vi "SpeakerTask.vi"(0 "stop":bool, 3 "ChanSelect":enum16{"Left", "Right", "Stereo"}(ring), 4 "path":path=path "E:/Code/Labview/SoundIdentity/Sounds/Test/TestANJALI.wav") -> (1 "Waveform Graph":waveform(dbl)[](graph)=[{"t0"=timestamp(0 s since 1904-01-01), "dt"=6.25e-05, "Y"=array[16640 elements]}])   [LabVIEW 2010]
doc: "I. Description:\nThis example demonstrates how to output a continuous periodic waveform using an internal sample clock.\n\nII. Instructions for Running:\n1. Select the Physical Channel to correspond to where your signal is output on the DAQ device.\n2. Enter the Minimum and Maximum Voltage Ranges\n3. Specify the Desired Frequency of the output Waveform\n4. Enter the Waveform Information. See the documentation of the Waveform Buffer Generation SubVI for information on each parameter.\n\nIII. Block Diagram Steps:\n1. Create an Analog Output Voltage channel.\n2. Call the DAQmx Timing (Use Waveform) VI which sets the sample clock rate based on the input waveform parameters, and set the sample mode to Continuous.\n3. Write the waveform to the output buffer.\n4. Call the Start VI.\n5. Loop continuously until the user presses the Stop button. Check for errors every 100 ms using the Is Task Done? VI\n6. Clear the Task\n7. Use the popup dialog box to display an error or warning if any.\n\nIV. I/O Connections Overview:\nMake sure your signal output terminal matches the Physical Channel I/O Control. For further connection information, refer to your hardware reference manual."
uses:
  <vilib>/Utility/error.llb/DialogType.ctl
  <vilib>/DAQmx/write.llb/DAQmx Write (Analog 2D DBL NChan NSamp).vi
  <vilib>/DAQmx/configure/timing.llb/DAQmx Timing (Sample Clock).vi
  <vilib>/measure/maspectr.llb/FFT Power Spectrum for N Chan.vi
  <vilib>/daqmx/miscellaneous.llb/DAQmx Fill In Error Info.vi
  <vilib>/DAQmx/create/channels.llb/DAQmx Create Channel (AO-Voltage-Basic).vi
  <vilib>/measure/NI_MAPro.lvlib
panel:
  in  "Power Spectrum":bool
  out "Power Spectrum 2":cluster{"f0":dbl, "df":dbl, "magnitude":dbl[]}[](graph)
  out "Done":bool=TRUE
  out "Completed":dbl=1.0 format="%0.0f"
  in  "restart":bool
  in  "dB":bool=TRUE
  in  "stop 2":bool
  in  "window":T1(ring)=enum."Hanning"
  in  "averaging parameters":T2={"averaging mode"=enum."No averaging", "weighting mode"=enum."Exponential", "number of averages"=10} {"number of averages" min=1}
  in  "Minimum Value":dbl=-10.0 format="%0.2f"
  in  "Maximum Value":dbl=10.0 format="%0.2f"
  # "Real-Time Spectral Measurements"
  # "Sampling Rate"
  # "Wav File"
  # "Channel Parameters"
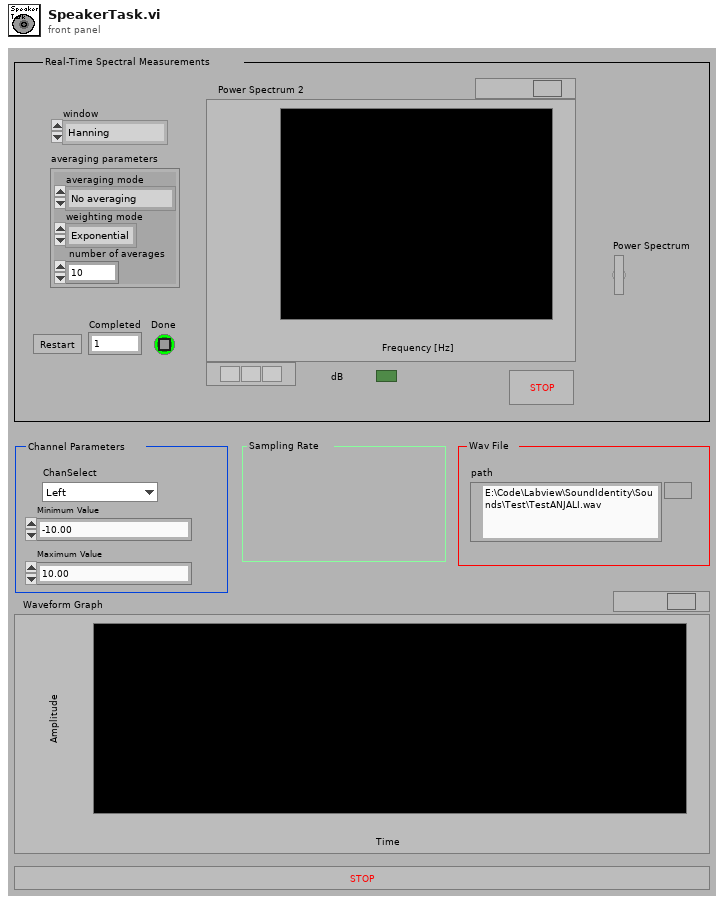
[diagram p1: front panel]
types:
  T1 = enum16{"None ", "Hanning", "Hamming", "Blackman-Harris", "Exact Blackman", "Blackman", "Flat Top", "4 Term B-Harris ", "7 Term B-Harris", "Low Sidelobe"}
  T2 = cluster{"averaging mode":enum16{"No averaging", "Vector averaging", "RMS averaging", "Peak hold"}, "weighting mode":enum16{"Linear", "Exponential"}, "number of averages":u32}
  T3 = typedef "DialogType.ctl" = u16
  T4 = cluster{"data[0]":waveform(dbl), "data[1]":waveform(dbl), "data[2]":waveform(dbl), "data[3]":waveform(dbl), "data[4]":waveform(dbl), "data[5]":waveform(dbl), "data[6]":waveform(dbl), "data[7]":waveform(dbl), "data[8]":waveform(dbl)}
  T5 = enum16{"Initialize", "String", "Start", "New Session", "Stop", "Resume", "Close"}
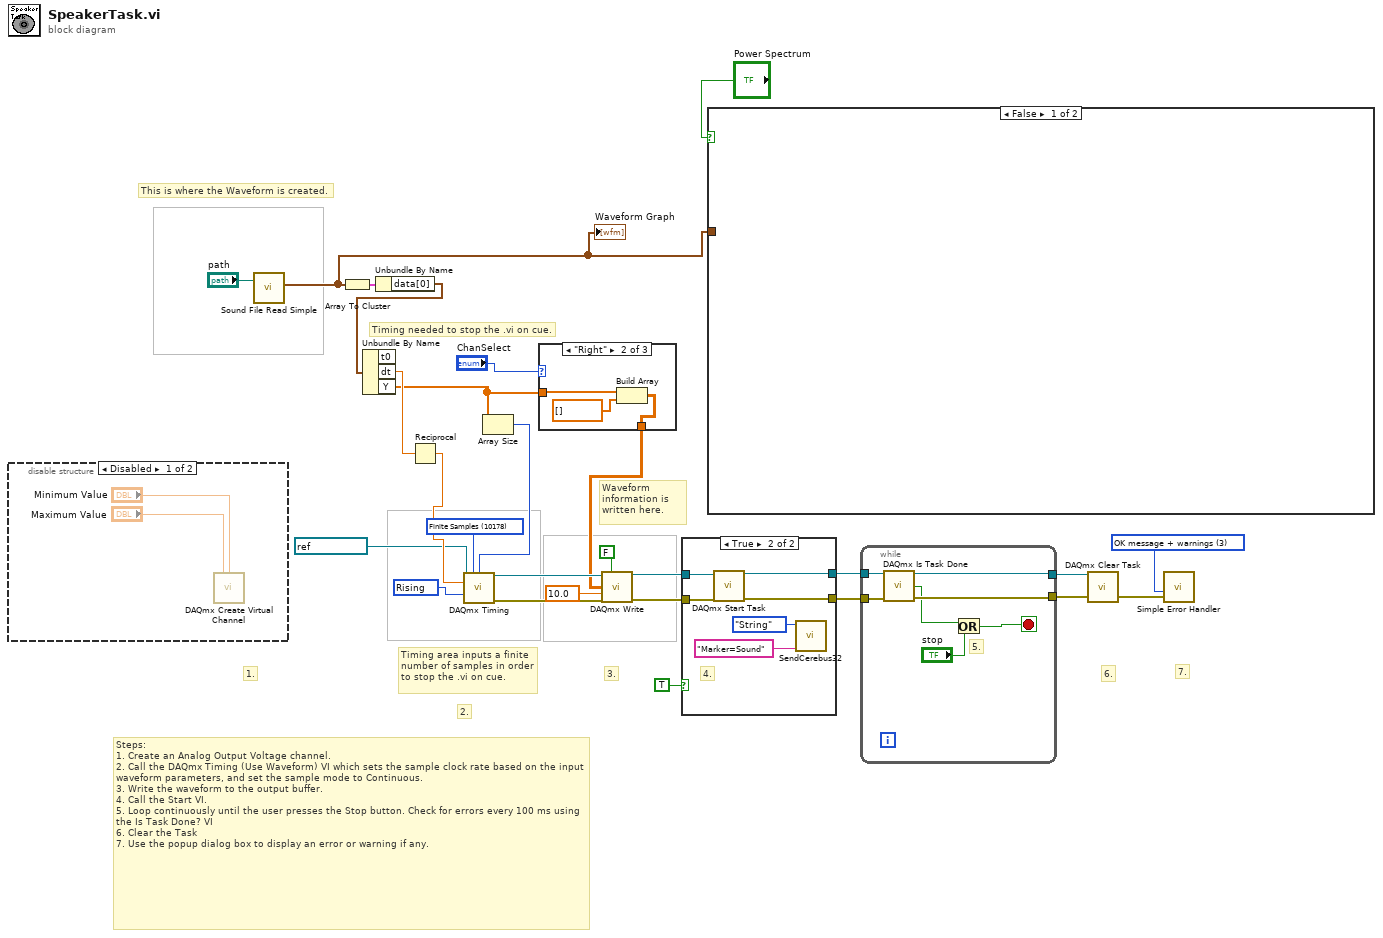
[diagram p0: block diagram]
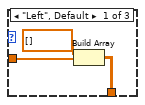
[diagram p2: hidden frame]
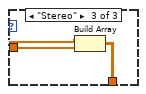
[diagram p3: hidden frame]
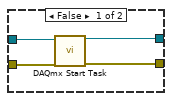
[diagram p5: hidden frame]
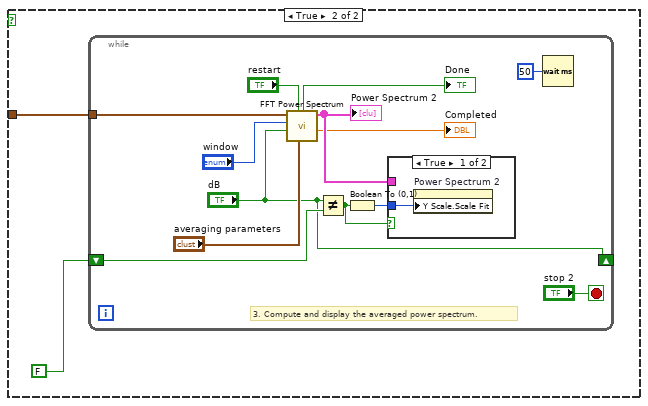
[diagram p6: hidden frame]
diagram:
  w15 = 10280 items=["Rising"=10280, "Falling"=10171] ("active edge")
  w18 = T3 3 items=["no dialog", "OK message", "continue or stop message", "OK message + warnings", "continue/stop + warnings"] ("type of dialog (OK msg:1)")
  w26 = 10178 items=["Finite Samples"=10178, "Continuous Samples"=10123] ("sample mode")
  # "Waveform information is written here."
  # "Timing area inputs a finite number of samples in order to stop the .vi on cue."
  # "Timing needed to stop the .vi on cue."
  # "This is where the Waveform is created."
  # "7."
  # "6."
  # "Steps: \n1. Create an Analog Output Voltage channel.\n2. Call the DAQmx Timing (Use Waveform) VI which sets the sample clock rate based on the input waveform parameters, and set the sample mode to Continuous.\n3. Write the waveform to the output buffer.\n4. Call the Start VI.\n5. Loop continuously until the user presses the Stop button. Check for errors every 100 ms using the Is Task Done? VI\n6. Clear the Task\n7. Use the popup dialog box to display an error or warning if any."
  # "3."
  # "2."
  # "1."
  n1 = disable-structure shown="Disabled" {
    frame Disabled {
      n2 = call-poly <vilib>:"DAQmx Create Virtual Channel.vi"("maximum value"="Maximum Value", "minimum value"="Minimum Value") -> ()  [unwired: 12 in, 2 out]
    }
    frame Enabled {
    }
  }
  n3 = call <vilib>:"Sound File Read Simple.vi"("path"="path") -> ("data"=w8:waveform(dbl)[])  [unwired: 7 in, 3 out]
  "Waveform Graph" <- w8
  n4 = Array To Cluster(array=w8) -> (cluster=w10:T4)
  n5 = Unbundle By Name(w10) -> ("data[0]"=w9:waveform(dbl))
  n6 = Unbundle By Name(w9) -> ("dt"=w6:dbl, "Y"=w3:dbl[])  [unwired: 1 out]
  n7 = Reciprocal(x=w6) -> (1/x=w5:dbl)
  n8 = Array Size(array=w3) -> (size(s)=w7:i32)
  n9 = call-poly <vilib>:"DAQmx Timing.vi"("task/channels in"=refnum<k21> "AudioOut", "sample mode"=w26, "samples per channel"=w7, "rate"=w5, "active edge"=w15) -> ("task out"=w21:refnum<k21>, "error out"=w20:errorcluster)  [unwired: 9 in]
  n10 = case shown="\"Right\"" "ChanSelect" {
    tunnel: w3 -> [w31 w34 w37]
    tunnel: [w32 w35 w36] -> w2
    frame "Left", Default {
      n11 = Build Array(dbl[] [] ("element"), w31) -> (w32:dbl[][])
    }
    frame "Right" {
      n12 = Build Array(w34, dbl[] [] ("element")) -> (w35:dbl[][])
    }
    frame "Stereo" {
      n13 = Build Array(w37, w37) -> (w36:dbl[][])
    }
  }
  n14 = call-poly <vilib>:"DAQmx Write.vi"("task/channels in"=w21, "auto start"=FALSE, "data"=w2, "timeout"=10.0 ("Wirite Timeout"), "error in"=w20) -> ("task out"=w25:refnum<k21>, "error out"=w24:errorcluster)  [unwired: 8 in, 1 out]
  n15 = case shown="True" TRUE {
    tunnel: w25 -> [w41 w47]
    tunnel: w24 -> [w40 w46]
    tunnel: [w38 w45] -> w22
    tunnel: [w39 w44] -> w19
    frame False {
      n16 = call <vilib>:"DAQmx Start Task.vi"("task/channels in"=w41, "error in"=w40) -> ("task out"=w39:refnum<k21>, "error out"=w38:errorcluster)  [unwired: 12 in]
    }
    frame True {
      # "4."
      n17 = call <vilib>:"DAQmx Start Task.vi"("task/channels in"=w47, "error in"=w46) -> ("task out"=w44:refnum<k21>, "error out"=w45:errorcluster)  [unwired: 12 in]
      n18 = call "SendCerebus32.vi"("String"="Marker=Sound" ("ASCII Data"), "Mode"=T5."String") -> ()  [unwired: 3 in]
    }
  }
  n19 = case shown="False" "Power Spectrum" {
    tunnel: w8 -> [_ w48]
    frame False {
    }
    frame True {
      n20 = while {
        shift-left: FALSE ("dB") -> [w56]
        shift-right: ["dB"] -> _
        tunnel: w48 -> [w50]
        stop <- "stop 2" stop-if-true
        # "3. Compute and display the averaged power spectrum."
        n21 = call-poly <vilib>:"FFT Power Spectrum.vi"("averaging parameters"="averaging parameters", "restart averaging (F)"="restart", "dB On (F)"="dB", "window"="window", "time signals"=w50) -> ("averages completed"=→"Completed":dbl, "power spectra"=w60:cluster{"f0":dbl, "df":dbl, "magnitude":dbl[]}[], "averaging done"=→"Done":bool)  [unwired: 3 in, 1 out]
        "Power Spectrum 2" <- w60
        n22 = Not Equal?(x="dB", y=w56) -> (x != y?=w55:bool)
        n23 = Boolean To (0,1)(Boolean=w55) -> (0, 1=w54:i16)
        n24 = case shown="True" w55 {
          tunnel: w54 -> [w63 _]
          tunnel: w60 -> [_ _]
          frame True {
            n25 = property on="Power Spectrum 2" class="WFGraph (strict)"("Y Scale.Scale Fit"=w63) -> ()  [unwired: 2 in, 2 out]
          }
          frame False {
          }
        }
        n26 = Wait (ms)(milliseconds to wait=u32 50 ("millisecond multiple")) -> ()  [unwired: 1 out]
      }
    }
  }
  n27 = while {
    tunnel: w19 -> [w70]
    tunnel: [w69] -> w17
    tunnel: w22 -> [w68]
    tunnel: [w67] -> w16
    stop <- w66 stop-if-true
    # "5."
    n28 = call <vilib>:"DAQmx Is Task Done.vi"("task/channels in"=w70, "error in"=w68) -> ("task out"=w69:refnum<k21>, "task done?"=w64:bool, "error out"=w67:errorcluster)  [unwired: 11 in]
    n29 = Or(x=w64, y="stop") -> (x .or. y?=w66:bool)
  }
  n30 = call <vilib>:"DAQmx Clear Task.vi"("task in"=w17, "error in"=w16) -> ("error out"=w27:errorcluster)  [unwired: 13 in]
  n31 = call <vilib>:"Simple Error Handler.vi"("type of dialog (OK msg:1)"=w18, "error in (no error)"=w27) -> ()  [unwired: 3 in, 5 out]
